vi "Load Parser Settings.vi"(8 "Error in":errorcluster caption="Error in (no error)", 11 "Settings Path":path) -> (0 "Error out":errorcluster, 1 "Loaded Default?":bool, 3 "Parser Settings":T1)   [LabVIEW 2023, in "VIDoc Parsing.lvlib" / "Parser Settings.lvclass"]
uses:
  Parser Settings.lvclass
  Parser Settings Cluster.ctl
  Draw Controls Cluster.ctl
  Draw Option Enum.ctl
  ac5b38ed-98c3-46aa-8a0e-3b9f0d21d897.vi
  <vilib>/JDP Science/JSONtext/JSON text to Variant.vi
  <vilib>/JDP Science/JSONtext/LVClass Serializer/JSONtext LVClass Serializer.lvclass
  VIDoc Settings/VIDoc Settings.lvclass
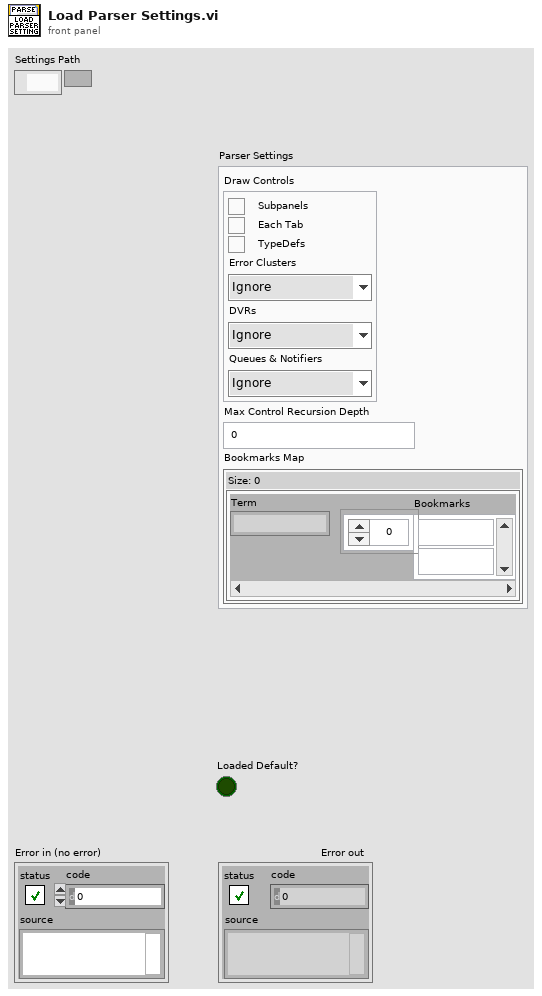
[diagram p1: front panel]
types:
  T1 = typedef "VIDoc Parsing.lvlib/Parser Settings.lvclass/Parser Settings Cluster.ctl" = cluster{"Draw Controls":T2, "Max Control Recursion Depth":i32, "Bookmarks Map":map{string, string[]}}
  T2 = typedef "VIDoc Parsing.lvlib/Parser Settings.lvclass/Draw Controls Cluster.ctl" = cluster{"Subpanels":bool, "Tabs":bool, "TypeDefs":bool, "Error Clusters":T3, "DVRs":T3, "Queues & Notifiers":T3}
  T3 = typedef "VIDoc Parsing.lvlib/Parser Settings.lvclass/Draw Option Enum.ctl" = enum16{"Ignore", "Draw", "Draw + Contents"}
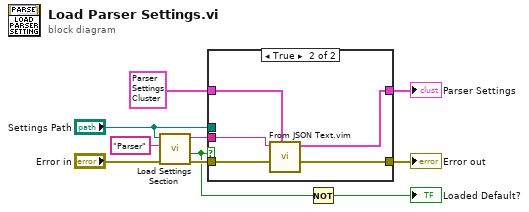
[diagram p0: block diagram]
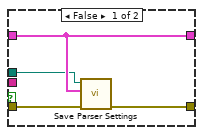
[diagram p2: hidden frame]
diagram:
  n1 = call "Load Settings Section.vi"("Error in"="Error in", "Section Name"="Parser", "JSON Settings Path"="Settings Path") -> ("Error out"=w8:errorcluster, "Found"=w2:bool, "JSON Object"=w7:string)  [unwired: 6 in]
  n2 = case shown="True" w2 {
    tunnel: w8 -> [w14 w19]
    tunnel: w7 -> [_ w18]
    tunnel: T1 {"Draw Controls"={"Subpanels"=TRUE, "Tabs"=TRUE, "TypeDefs"=TRUE, "Error Clusters"=enum."Draw", "DVRs"=enum."Draw", "Queues & Notifiers"=enum."Draw"}, "Max Control Recursion Depth"=10, "Bookmarks Map"={}} ("Parser Settings") -> [w12 w17]
    tunnel: [w12 w16] -> w5
    tunnel: [w13 w15] -> w4
    tunnel: "Settings Path" -> [w11 _]
    frame False {
      n3 = call "Save Parser Settings.vi"("Error in"=w14, "Parser Settings"=w12, "Settings Path"=w11) -> ("Error out"=w13:errorcluster)  [unwired: 8 in]
    }
    frame True {
      n4 = call "From JSON Text.vim"("Data Type and Default Value"=w17, "error in (no error)"=w19, "JSON"=w18) -> ("error out"=w15:errorcluster, "Data out"=w16:T1)  [unwired: 7 in]
    }
  }
  "Error out" <- w4
  "Parser Settings" <- w5
  n5 = Not(x=w2) -> (.not. x?=→"Loaded Default?":bool)
